vi "Update Log Start Time if New Trigger.vi"(9 "Previous Trigger Value":i32, 10 "Current Trigger Value":i32, 11 "Previous Log Trigger Time":timestamp) -> (3 "Current Log Trigger Time":timestamp)   [LabVIEW 2027, in "Embedded Data Logger Engine.lvlib"]
uses:
  Embedded Data Logger Engine.lvlib
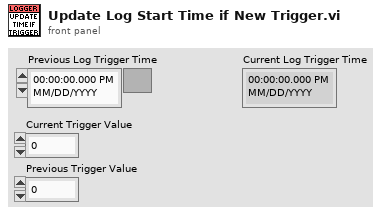
[diagram p1: front panel]
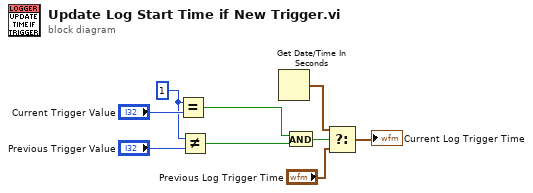
[diagram p0: block diagram]
diagram:
  w5 = 1 ("y")
  n1 = Equal?(x=w5, y="Current Trigger Value") -> (x = y?=w9:bool)
  n2 = Not Equal?(x=w5, y="Previous Trigger Value") -> (x != y?=w4:bool)
  n3 = Get Date/Time In Seconds() -> (seconds since 1Jan1904=w3:timestamp)
  n4 = And(x=w9, y=w4) -> (x .and. y?=w8:bool)
  n5 = Select(t=w3, s=w8, f="Previous Log Trigger Time") -> (s? t:f=→"Current Log Trigger Time":timestamp)
